vi "GetTerminalUID.vi"(6 "error in":errorcluster, 9 "Tunnel in":refnum<class "Tunnel.lvclass">) -> (0 "error out":errorcluster, 3 "Tunnel out":refnum<class "Tunnel.lvclass">, 4 "outer terminal UID":i32, 5 "inner terminal UIDs":i32[](array[numeric]))   [LabVIEW 2014, in "Tunnel.lvclass"]
uses:
  Tunnel.lvclass
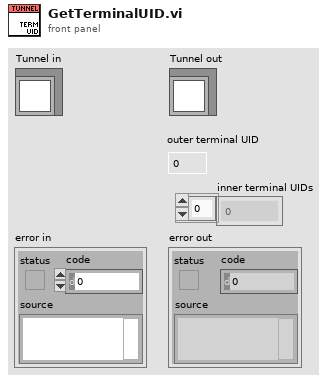
[diagram p1: front panel]
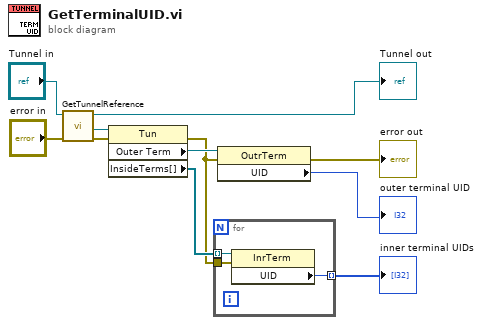
[diagram p0: block diagram]
diagram:
  n1 = call "GetTunnelReference.vi"("error in"="error in", "Tunnel in"="Tunnel in") -> ("error out"=w8:errorcluster, "reference out"=w7:refnum<vi>, "Tunnel out"=→"Tunnel out":refnum<class "Tunnel.lvclass">)  [unwired: 7 in]
  n2 = property class="Tun"(reference=w7, error in=w8) -> (error out=w2:errorcluster, "Outer Term"=w11:refnum<vi>, "InsideTerms[]"=w3:refnum<vi>[])  [unwired: 1 out]
  n3 = for {
    tunnel: w3 -> [w14] mode=indexing
    tunnel: [w13] -> w1 mode=indexing
    tunnel: w2 -> [w12]
    n4 = property class="InrTerm"(reference=w14, error in=w12) -> ("UID"=w13:i32)  [unwired: 2 out]
  }
  "inner terminal UIDs" <- w1
  n5 = property class="OutrTerm"(reference=w11, error in=w2) -> (error out=→"error out":errorcluster, "UID"=→"outer terminal UID":i32)  [unwired: 1 out]
